vi "Prevent over max lines.vi"(0 "Existing number of lines across all ROI":i32, 1 "Modify":bool, 5 "Array in":T1[](array[typedef]) {"Apparent Frame Size" format="%#_6f"; "Original FOV (um)" format="%#_6f"; "Pixels per miniscan" format="%#_6f"; "Dwell Time per pixel" format="%#_6f"; "Resolution" format="%#_6f"; "ROI group ID" format="%#_6f"; "Laser Power (%)" format="%#_6f"; "Zoom" format="%#_6f"; "Frame Size" format="%#_6f"; "Number of lines" format="%#_6f"; "Composite ID" format="%#_6f"; "Angle (deg)" format="%#_6f"; "ROI Time (ns)" format="%#_6f"; "ROI ID" format="%#_6f"; "Pixels in ROI" format="%#_6f"; "ROI index" format="%#_6f"; "Z stop" format="%#_6f"; "Y stop" format="%#_6f"; "X stop" format="%#_6f"; "Z start" format="%#_6f"; "X start" format="%#_6f"; "Y start" format="%#_6f"}, 7 "Mod. ROI Idx":i32, 9 "X-Y-Z coordinates":T1 {"Apparent Frame Size" format="%#_6f"; "Original FOV (um)" format="%#_6f"; "Pixels per miniscan" format="%#_6f"; "Dwell Time per pixel" format="%#_6f"; "Resolution" format="%#_6f"; "ROI group ID" format="%#_6f"; "Laser Power (%)" format="%#_6f"; "Zoom" format="%#_6f"; "Frame Size" format="%#_6f"; "Number of lines" format="%#_6f"; "Composite ID" format="%#_6f"; "Angle (deg)" format="%#_6f"; "ROI Time (ns)" format="%#_6f"; "ROI ID" format="%#_6f"; "Pixels in ROI" format="%#_6f"; "ROI index" format="%#_6f"; "Z stop" format="%#_6f"; "Y stop" format="%#_6f"; "X stop" format="%#_6f"; "Z start" format="%#_6f"; "X start" format="%#_6f"; "Y start" format="%#_6f"}, 11 "New number of lines to be added (1)":i32=1, 12 "Number of ROI":i32) -> (3 "Hardware limitation (number of lines across al ROI)":i32=1024, 4 "Resulting number of lines across all ROI":i32, 6 "Array out":T1[](array[typedef]) {"Apparent Frame Size" format="%#_6f"; "Original FOV (um)" format="%#_6f"; "Pixels per miniscan" format="%#_6f"; "Dwell Time per pixel" format="%#_6f"; "Resolution" format="%#_6f"; "ROI group ID" format="%#_6f"; "Laser Power (%)" format="%#_6f"; "Zoom" format="%#_6f"; "Frame Size" format="%#_6f"; "Number of lines" format="%#_6f"; "Composite ID" format="%#_6f"; "Angle (deg)" format="%#_6f"; "ROI Time (ns)" format="%#_6f"; "ROI ID" format="%#_6f"; "Pixels in ROI" format="%#_6f"; "ROI index" format="%#_6f"; "Z stop" format="%#_6f"; "Y stop" format="%#_6f"; "X stop" format="%#_6f"; "Z start" format="%#_6f"; "X start" format="%#_6f"; "Y start" format="%#_6f"}, 8 "Modified/Added":bool, 10 "Exceeded 1024 lines":bool, 14 "Number of ROI":i32)   [LabVIEW 2020]
uses:
  User Interface/Visualisation/Functional Imaging Viewer/Typedefs/ROI parameters data type.ctl
  Typedefs/ROI ID Enum.ctl
  Global Variables/General Globals.vi
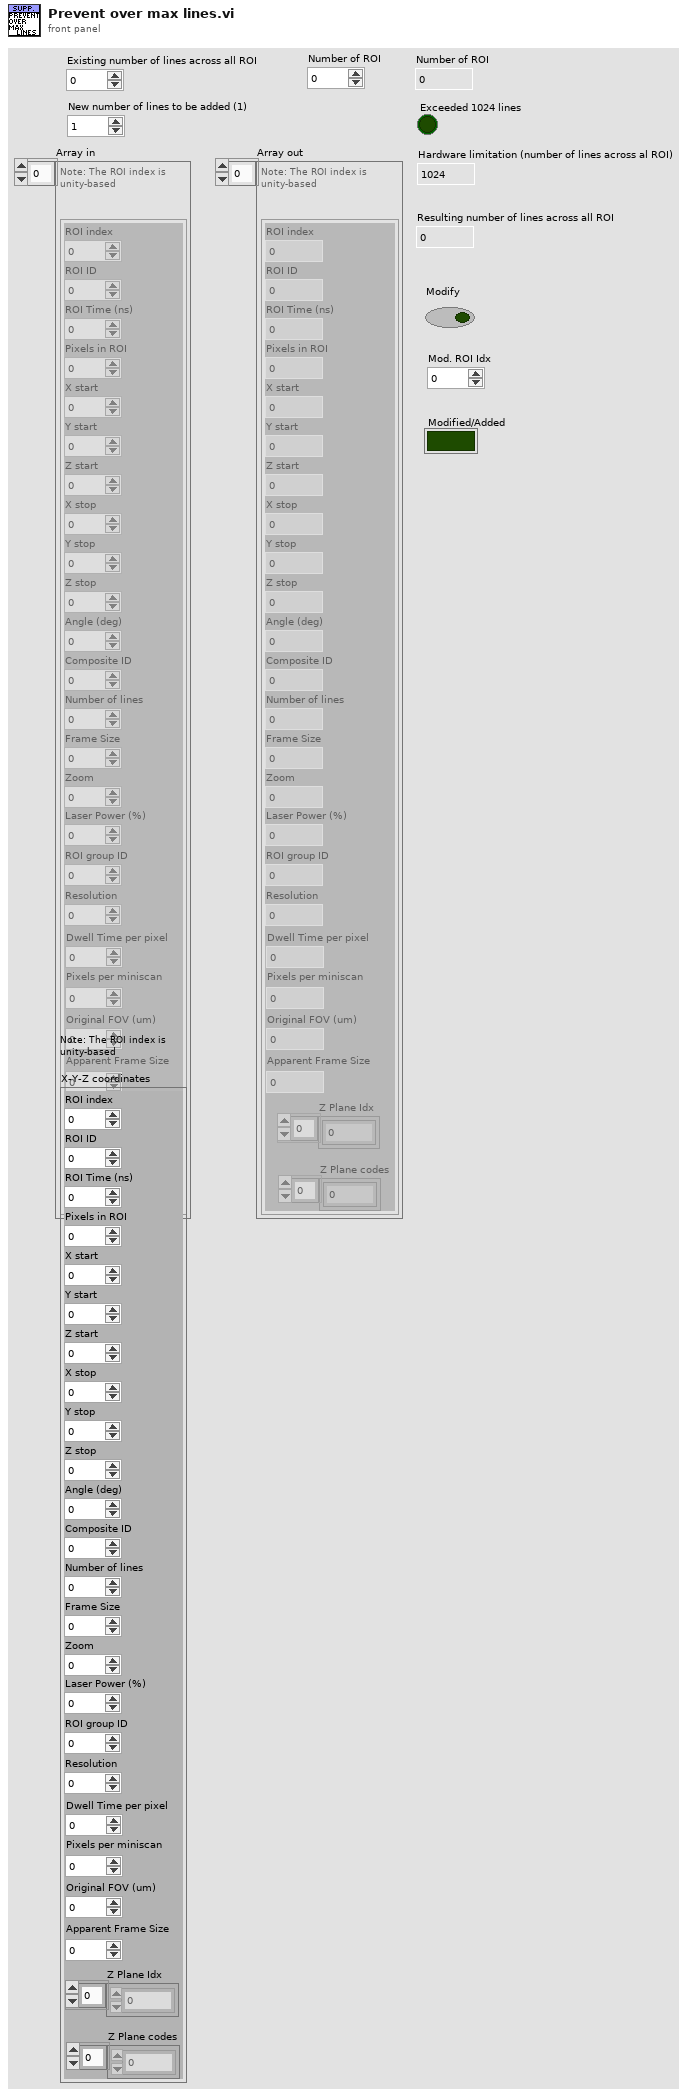
[diagram p1: front panel]
types:
  T1 = typedef "ROI parameters data type.ctl" = cluster{"ROI index":dbl, "ROI ID":dbl, "ROI Time (ns)":dbl, "Pixels in ROI":dbl, "X start":dbl, "Y start":dbl, "Z start":dbl, "X stop":dbl, "Y stop":dbl, "Z stop":dbl, "Angle (deg)":dbl, "Composite ID":dbl, "Number of lines":dbl, "Frame Size":dbl, "Zoom":dbl, "Laser Power (%)":dbl, "ROI group ID":dbl, "Resolution":dbl, "Dwell Time per pixel":dbl, "Pixels per miniscan":dbl, "Original FOV (um)":dbl, "Apparent Frame Size":dbl, "Z Plane Idx":i32[], "Z Plane codes":i32[]}
  T2 = typedef "ROI ID Enum.ctl" = enum16{"Point", "MiniScan", "Comp. MiniScan", "Rectangle", "Comp. volume", "Arb. plane point", "None"}
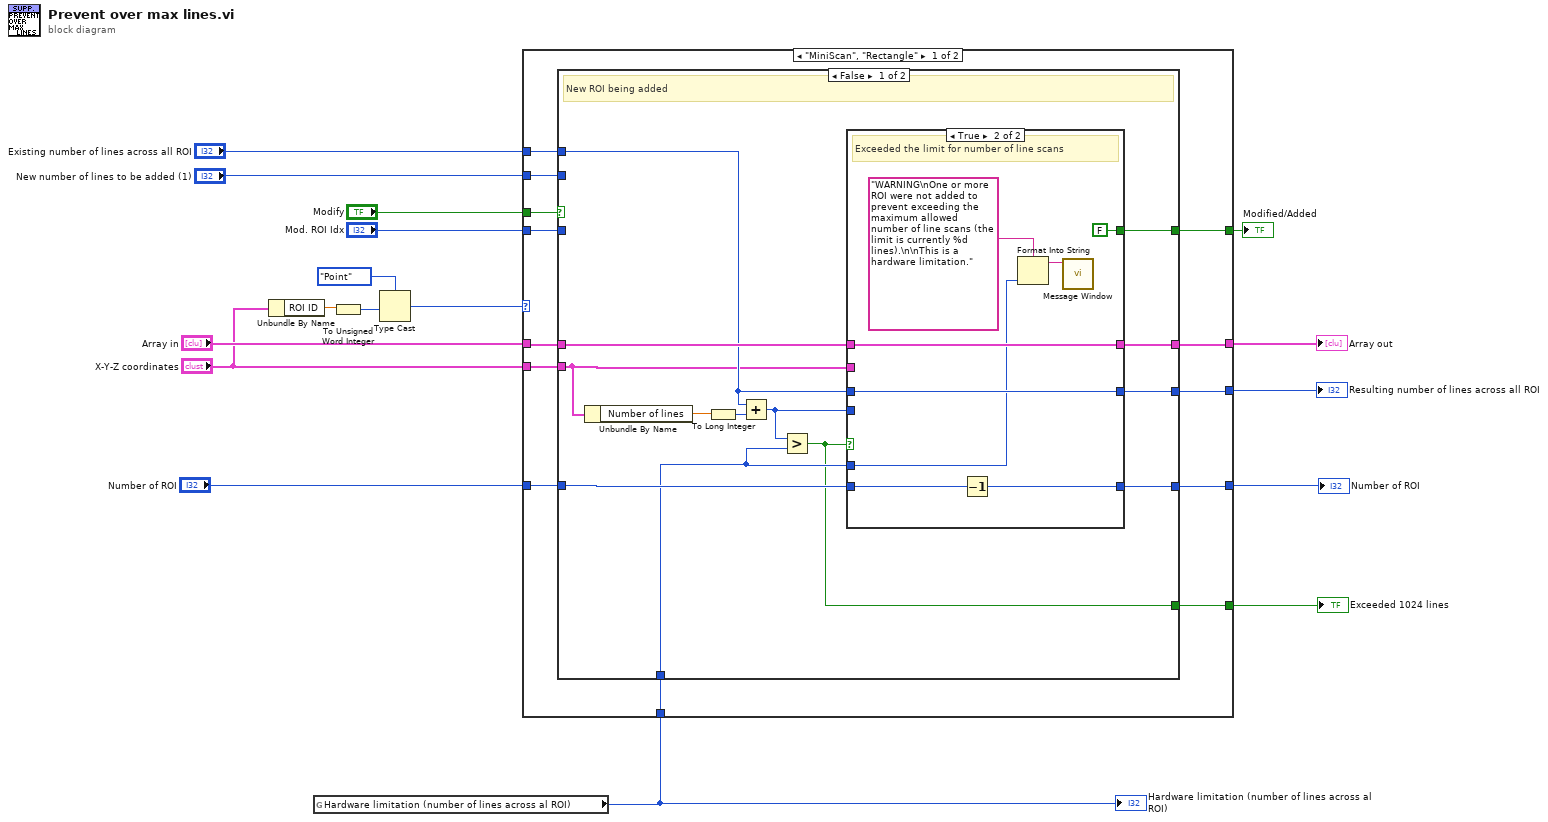
[diagram p0: block diagram]
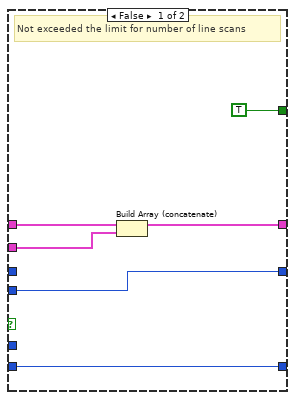
[diagram p2: hidden frame]
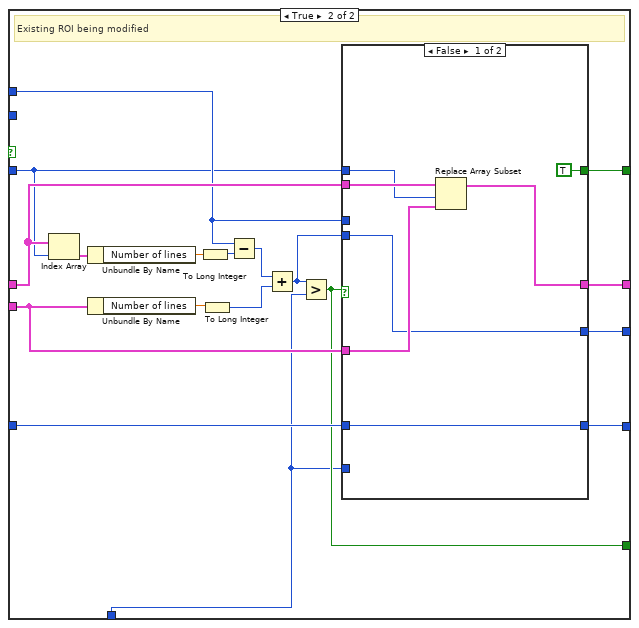
[diagram p3: hidden frame]
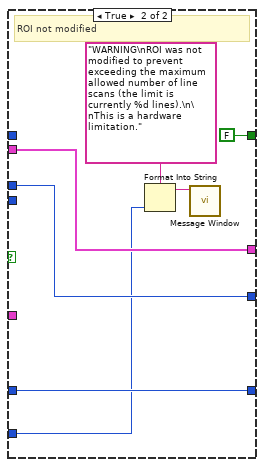
[diagram p4: hidden frame]
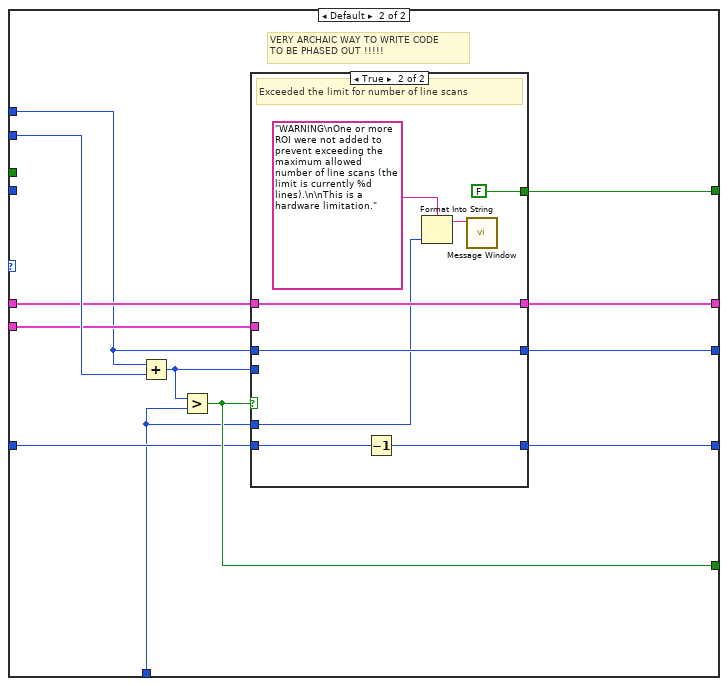
[diagram p5: hidden frame]
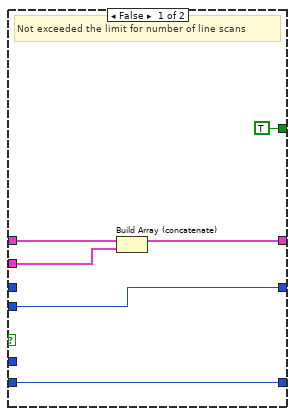
[diagram p6: hidden frame]
diagram:
  n1 = Unbundle By Name("X-Y-Z coordinates") -> ("ROI ID"=w7:dbl)
  n2 = global read "General Globals.vi" "Hardware limitation (number of lines across al ROI)"() -> (w9:i32)
  "Hardware limitation (number of lines across al ROI)" <- w9
  n3 = To Unsigned Word Integer(number=w7) -> (unsigned 16bit integer=w6:u16)
  n4 = Type Cast(type=ROI_ID_Enum."Point" ("ROI Type"), x=w6) -> (*(type *) &x=w4:T2)
  n5 = case shown="\"MiniScan\", \"Rectangle\"" w4 {
    tunnel: "New number of lines to be added (1)" -> [w26 w101]
    tunnel: [w22 w100] -> w16
    tunnel: "Array in" -> [w29 w99]
    tunnel: [w21 w98] -> w14
    tunnel: "X-Y-Z coordinates" -> [w28 w97]
    tunnel: "Existing number of lines across all ROI" -> [w27 w96]
    tunnel: [w20 w95] -> w12
    tunnel: "Number of ROI" -> [w25 w93]
    tunnel: [w19 w92] -> w10
    tunnel: w9 -> [w23 w91]
    tunnel: "Modify" -> [w30 _]
    tunnel: "Mod. ROI Idx" -> [w24 _]
    tunnel: [w18 w90] -> w1
    frame "MiniScan", "Rectangle" {
      n6 = case shown="False" w30 {
        tunnel: w29 -> [w42 w69]
        tunnel: w28 -> [w33 w68]
        tunnel: w27 -> [w41 w66]
        tunnel: w26 -> [_ _]
        tunnel: w25 -> [w40 w64]
        tunnel: w24 -> [_ w62]
        tunnel: w23 -> [w39 w59]
        tunnel: [w38 w60] -> w22
        tunnel: [w37 w67] -> w21
        tunnel: [w36 w65] -> w20
        tunnel: [w35 w63] -> w19
        tunnel: [w34 w58] -> w18
        frame False {
          # "New ROI being added"
          n7 = Unbundle By Name(w33) -> ("Number of lines"=w32:dbl)
          n8 = To Long Integer(number=w32) -> (32bit integer=w31:i32)
          n9 = Add(x=w41, y=w31) -> (x+y=w43:i32)
          n10 = Greater?(x=w43, y=w39) -> (0:w38:bool)
          n11 = case shown="True" w38 {
            tunnel: w42 -> [w49 w57]
            tunnel: [w48 w57] -> w37
            tunnel: w33 -> [w47 _]
            tunnel: w41 -> [_ w56]
            tunnel: [w46 w56] -> w36
            tunnel: w43 -> [w46 _]
            tunnel: w40 -> [w45 w55]
            tunnel: [w45 w54] -> w35
            tunnel: w39 -> [_ w51]
            tunnel: [TRUE FALSE] -> w34
            frame False {
              # "Not exceeded the limit for number of line scans"
              n12 = Build Array (concatenate)(w49, w47) -> (w48:T1[])
            }
            frame True {
              # "Exceeded the limit for number of line scans"
              n13 = Decrement(x=w55) -> (x-1=w54:i32)
              n14 = Format Into String(format string="WARNING\nOne or more ROI were not added to prevent exceeding the maximum allowed number of line scans (the limit is currently %d lines).\n\nThis is a hardware limitation." ("message"), w51) -> (resulting string=w52:string)  [unwired: 2 in, 1 out]
              n15 = call "Message Window.vi"("Message string"=w52) -> ()  [unwired: 10 in, 1 out]
            }
          }
        }
        frame True {
          # "Existing ROI being modified"
          n16 = Index Array(array=w69, index=w62) -> (element=w74:T1)
          n17 = Unbundle By Name(w74) -> ("Number of lines"=w73:dbl)
          n18 = Unbundle By Name(w68) -> ("Number of lines"=w75:dbl)
          n19 = To Long Integer(number=w73) -> (32bit integer=w72:i32)
          n20 = To Long Integer(number=w75) -> (32bit integer=w70:i32)
          n21 = Subtract(x=w66, y=w72) -> (x-y=w71:i32)
          n22 = Add(x=w71, y=w70) -> (x+y=w61:i32)
          n23 = Greater?(x=w61, y=w59) -> (0:w60:bool)
          n24 = case shown="False" w60 {
            tunnel: w69 -> [w82 w87]
            tunnel: w68 -> [w80 _]
            tunnel: [w79 w87] -> w67
            tunnel: w66 -> [_ w86]
            tunnel: [w78 w86] -> w65
            tunnel: w64 -> [w77 w85]
            tunnel: [w77 w85] -> w63
            tunnel: w62 -> [w81 _]
            tunnel: w61 -> [w78 _]
            tunnel: w59 -> [_ w84]
            tunnel: [TRUE FALSE] -> w58
            frame False {
              n25 = Replace Array Subset(array=w82, new element=w80, index=w81) -> (w79:T1[])
            }
            frame True {
              # "ROI not modified"
              n26 = Format Into String(format string="WARNING\nROI was not modified to prevent exceeding the maximum allowed number of line scans (the limit is currently %d lines).\n\nThis is a hardware limitation." ("message"), w84) -> (resulting string=w88:string)  [unwired: 2 in, 1 out]
              n27 = call "Message Window.vi"("Message string"=w88) -> ()  [unwired: 10 in, 1 out]
            }
          }
        }
      }
    }
    frame Default {
      # "VERY ARCHAIC WAY TO WRITE CODE\nTO BE PHASED OUT !!!!!"
      n28 = Add(x=w96, y=w101) -> (x+y=w94:i32)
      n29 = Greater?(x=w94, y=w91) -> (0:w100:bool)
      n30 = case shown="True" w100 {
        tunnel: w99 -> [w107 w115]
        tunnel: [w106 w115] -> w98
        tunnel: w97 -> [w105 _]
        tunnel: w96 -> [_ w114]
        tunnel: [w104 w114] -> w95
        tunnel: w94 -> [w104 _]
        tunnel: w93 -> [w103 w113]
        tunnel: [w103 w112] -> w92
        tunnel: w91 -> [_ w109]
        tunnel: [TRUE FALSE] -> w90
        frame False {
          # "Not exceeded the limit for number of line scans"
          n31 = Build Array (concatenate)(w107, w105) -> (w106:T1[])
        }
        frame True {
          # "Exceeded the limit for number of line scans"
          n32 = Decrement(x=w113) -> (x-1=w112:i32)
          n33 = Format Into String(format string="WARNING\nOne or more ROI were not added to prevent exceeding the maximum allowed number of line scans (the limit is currently %d lines).\n\nThis is a hardware limitation." ("message"), w109) -> (resulting string=w110:string)  [unwired: 2 in, 1 out]
          n34 = call "Message Window.vi"("Message string"=w110) -> ()  [unwired: 10 in, 1 out]
        }
      }
    }
  }
  "Array out" <- w14
  "Exceeded 1024 lines" <- w16
  "Resulting number of lines across all ROI" <- w12
  "Number of ROI" <- w10
  "Modified/Added" <- w1
